vi "ConvertDocxToMDUsingWritage.vi"() -> ()   [LabVIEW 2018]
uses:
  <vilib>/regexp/Match Regular Expression.xnode
panel:
  out "FigureLabelForLink":string[](array[string])
  out "FinalOutput":string
  out "FiguresNumbers":string[](array[string])
  out "String":string
  in  "file path (use dialog)":path=path "C:/Users/jgsaenz/gitRepos/HMIComputers_documentation/00 Structure/LSST_HMI_SoftwareDocumentation_0_Structure.md"
  # "This VI mus be used after saving the docx file as md using the writage tool"
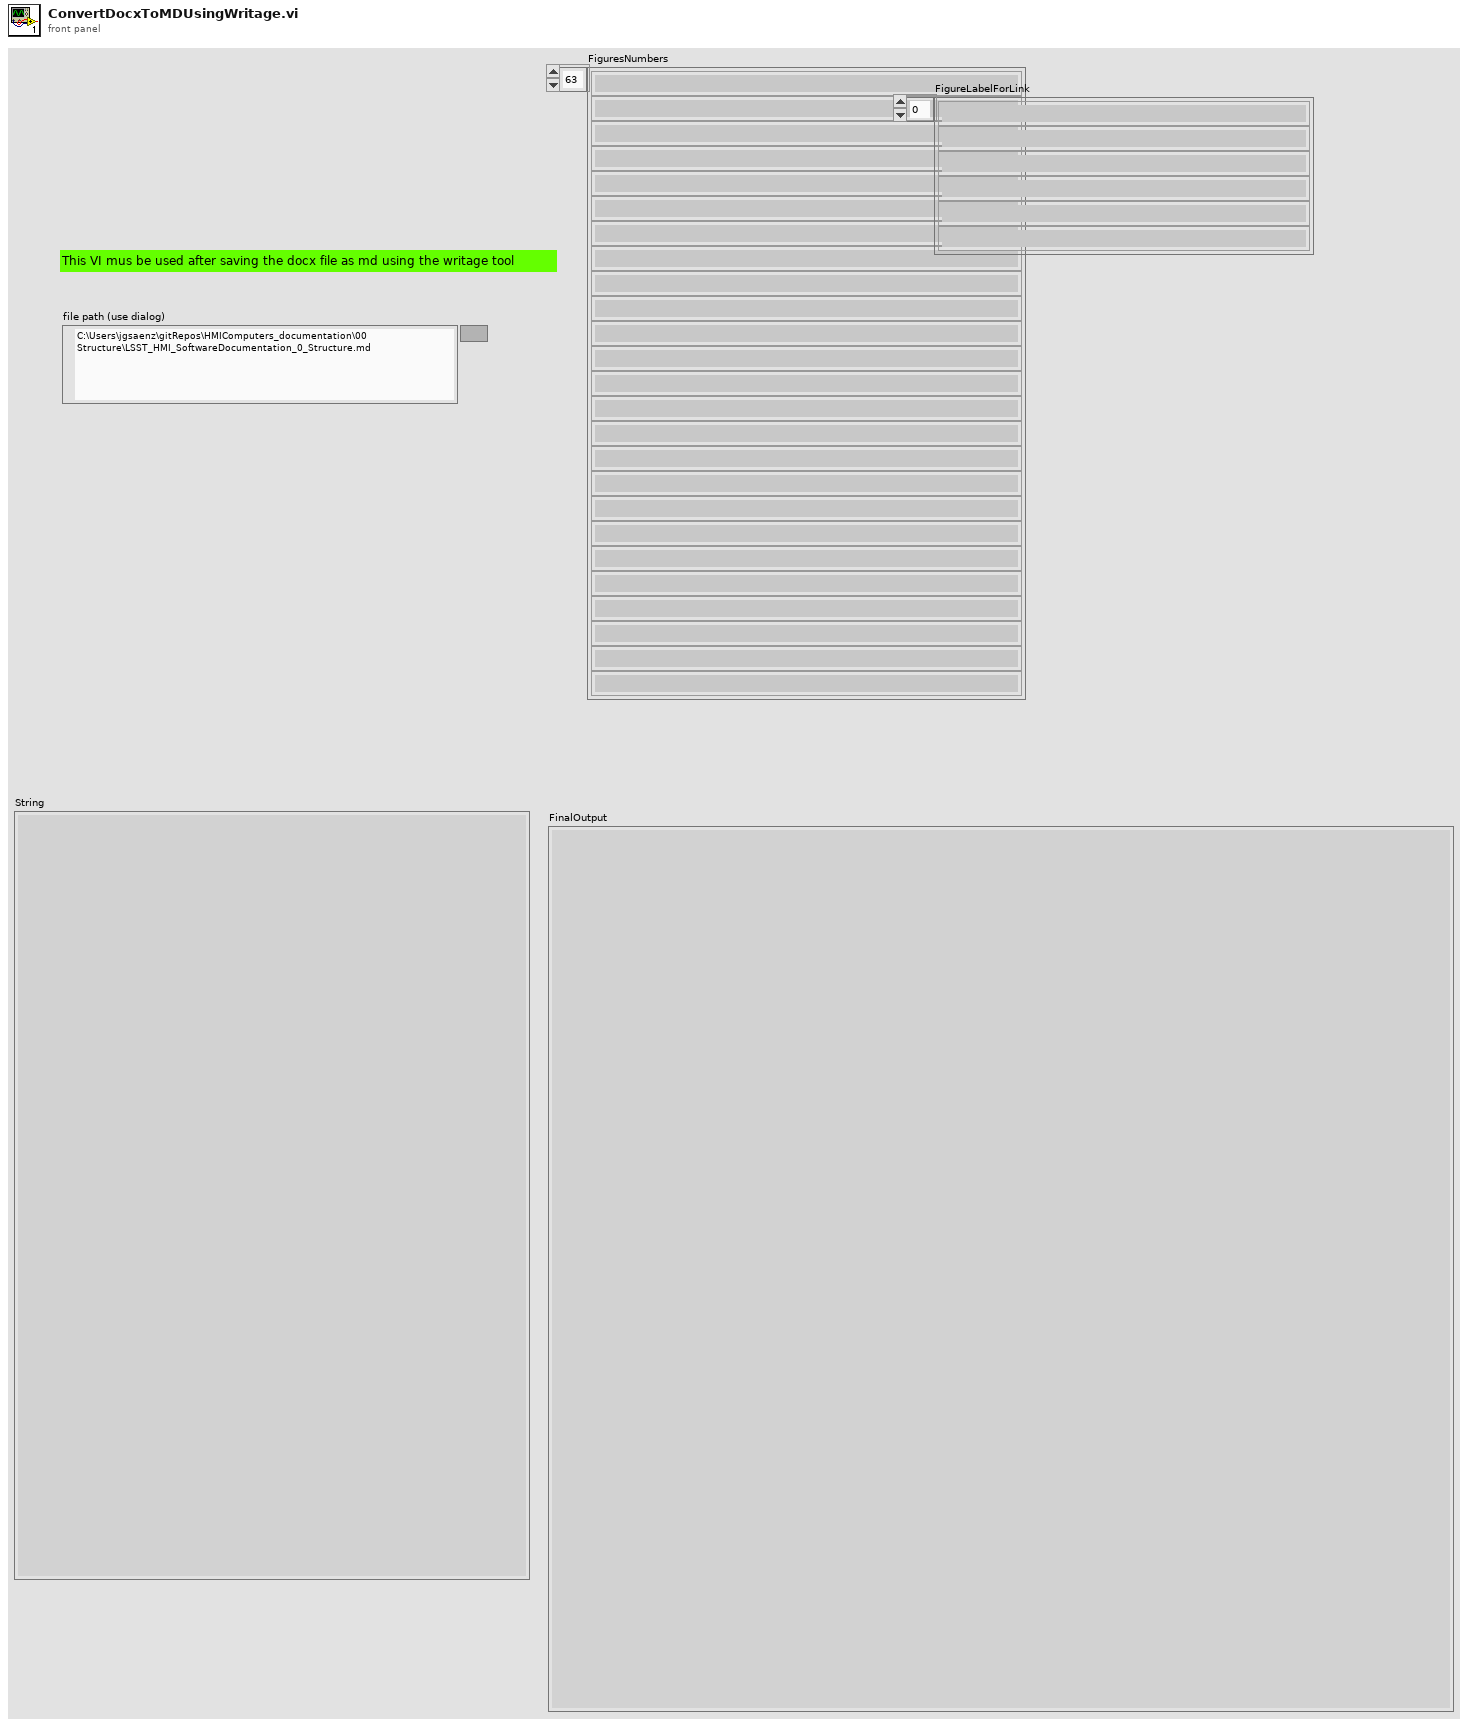
[diagram p1: front panel]
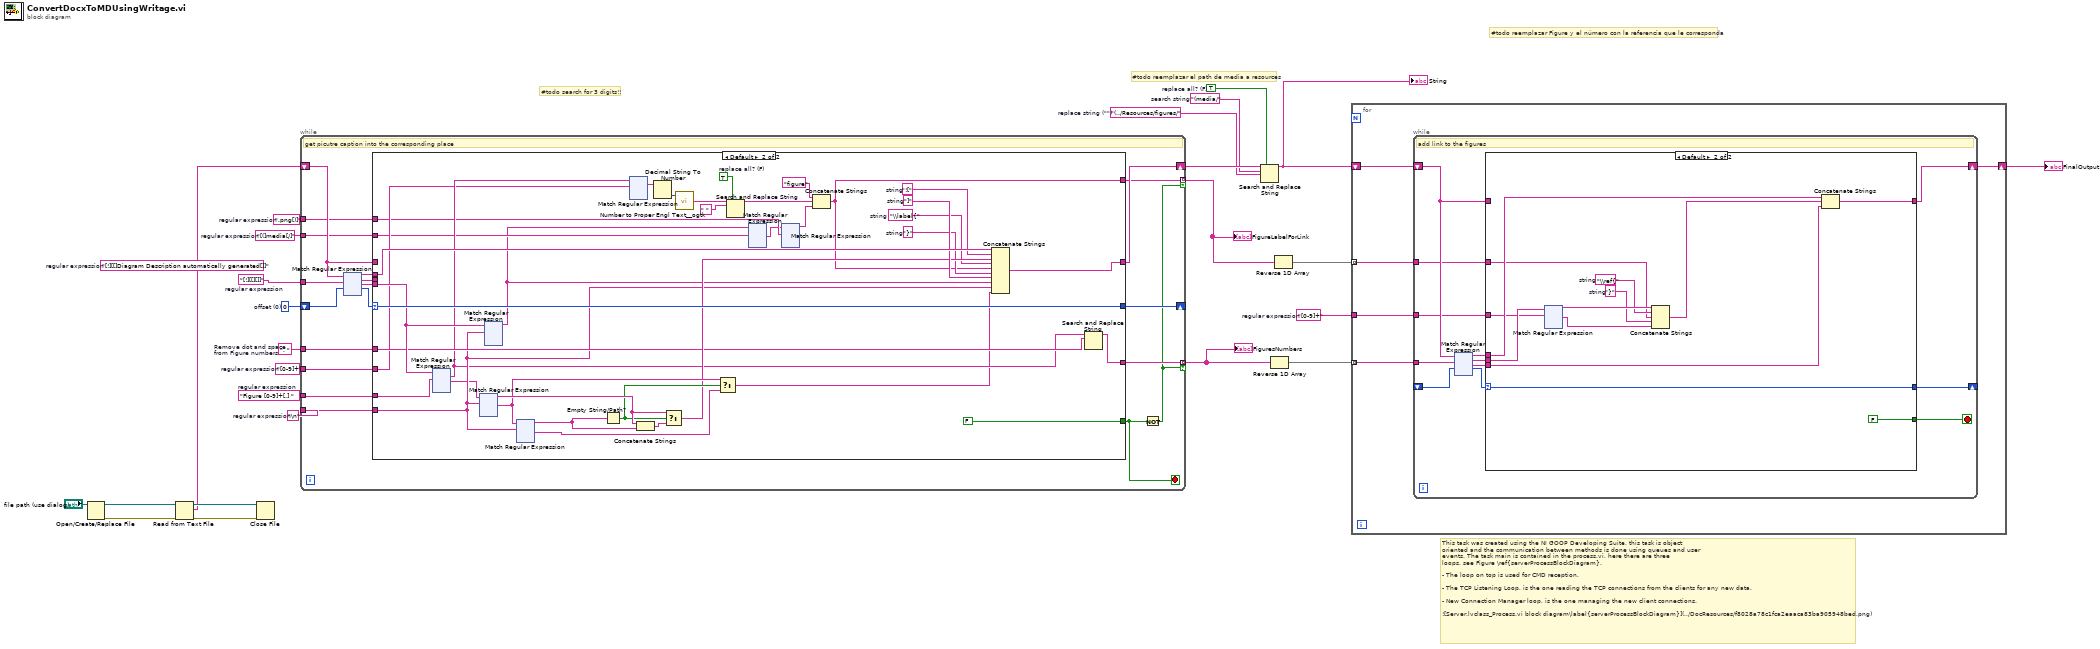
[diagram p0: block diagram]
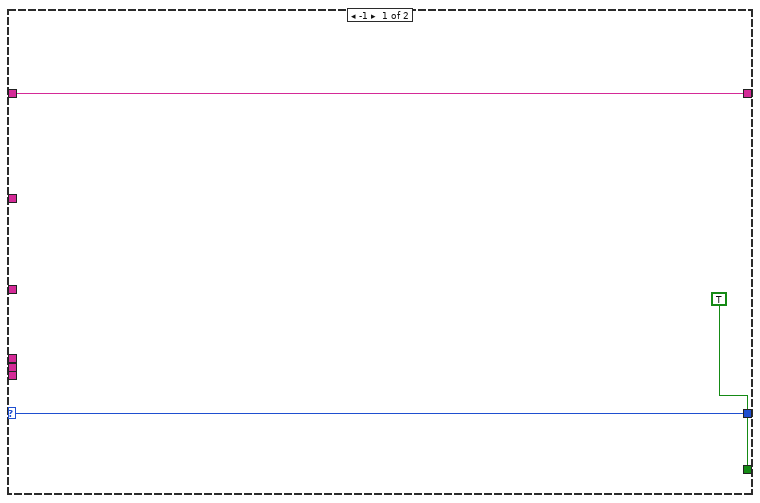
[diagram p2: hidden frame]
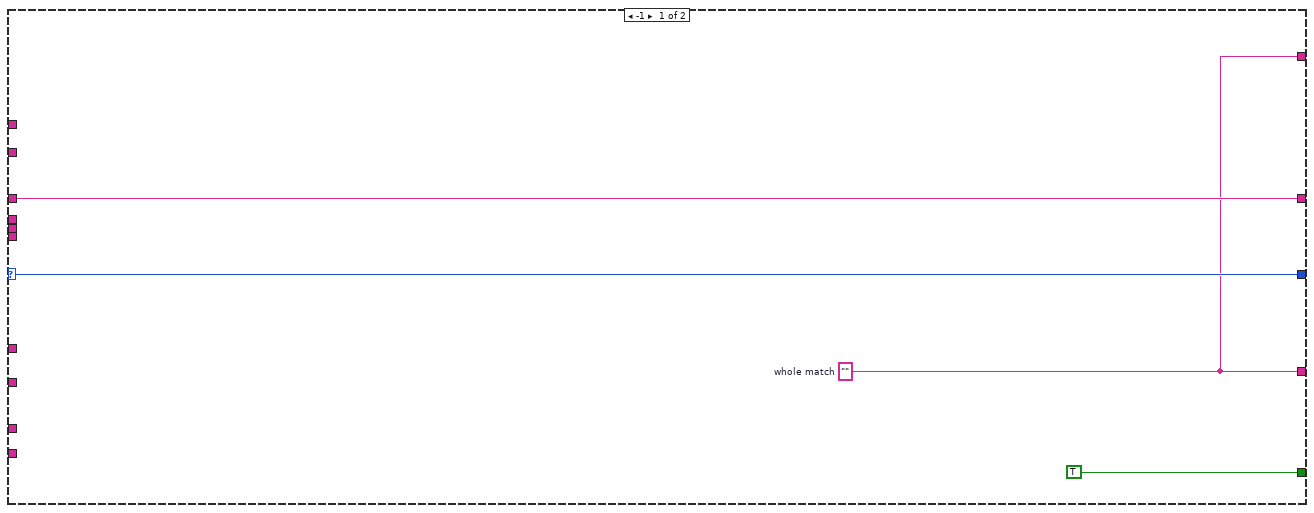
[diagram p3: hidden frame]
diagram:
  w3 = "[!][[][]]"  # regular expression
  w5 = "[0-9]+"  # regular expression
  w6 = TRUE  # replace all? (F)
  w7 = "[(]media[/]"  # regular expression
  w8 = ".png[)]"  # regular expression
  w9 = "[0-9]+"  # regular expression
  w10 = ". "  # Remove dot and space from Figure numbers
  w14 = "(../Resources/figures/"  # replace string ("")
  w15 = "(media/"  # search string
  w17 = 0  # offset (0)
  w18 = "\n"  # regular expression
  w19 = "Figure [0-9]+[.] "  # regular expression
  (unwired) "[!][[]Diagram Description automatically generated[]]"  # regular expression
  # "#todo search for 3 digits!!"
  # "#todo reemplazar el path de media a resources"
  # "#todo reemplazar Figure y el número con la referencia que le corresponda"
  # "This task was created using the NI GOOP Developing Suite, this task is object\noriented and the communication between methods is done using queues and user\nevents. The task main is contained in the process.vi, here there are three\nloops, see Figure \\ref{serverProcessBlockDiagram}.\n\n- The loop on top is used for CMD reception.\n\n- The TCP Listening Loop, is the one reading the TCP connections from the clients for any new data.\n\n- New Connection Manager loop, is the one managing the new client connections.\n\n![Server.lvclass_Process.vi block diagram\\label{serverProcessBlockDiagram}](../DocResources/f8028a78c1fca2eaaca83ba905948bed.png)"
  n1 = Open/Create/Replace File(file path (use dialog)="file path (use dialog)") -> (refnum out=w24:refnum<file>, error out=w25:errorcluster)  [unwired: 5 in, 1 out]
  n2 = Read from Text File(file (use dialog)=w24, error in=w25) -> (refnum out=w22:refnum<file>, text=w20:string, error out=w23:errorcluster)  [unwired: 2 in, 1 out]
  n3 = Close File(refnum=w22, error in=w23) -> ()  [unwired: 2 out]
  n4 = while {
    tunnel: w3 -> [w44]
    tunnel: w19 -> [w43]
    tunnel: w18 -> [w41]
    shift-right: [w38] -> _
    shift-left: w17 -> [w40]
    shift-right: [w36] -> w16
    shift-left: w20 -> [w37]
    tunnel: [w33] -> w11 mode=indexing if=w28
    tunnel: w10 -> [w31]
    tunnel: w9 -> [w30]
    tunnel: [w29] -> w4 mode=indexing if=w28
    tunnel: w8 -> [w27]
    tunnel: w7 -> [w26]
    stop <- w32 stop-if-true
    # "get picutre caption into the corresponding place"
    n5 = xnode "Match Regular Expression"("input string"=w37, "regular expression"=w44, "offset (0)"=w40) -> ("before match"=w34:string, "whole match"=w35:string, "after match"=w42:string, "offset past match"=w39:i32)  [unwired: 3 in, 1 out]
    n6 = case shown="Default" w39 {
      selector: w39 -> [w48 w81]
      tunnel: w43 -> [_ w85]
      tunnel: w42 -> [_ w75]
      tunnel: w41 -> [_ w66]
      tunnel: [w48 w81] -> w38
      tunnel: w37 -> [w47 _]
      tunnel: [w47 w79] -> w36
      tunnel: w35 -> [_ _]
      tunnel: w34 -> [_ w80]
      tunnel: [TRUE FALSE] -> w32
      tunnel: [w45 w70] -> w33
      tunnel: w31 -> [_ w69]
      tunnel: w30 -> [_ w62]
      tunnel: [w45 w60] -> w29
      tunnel: w27 -> [_ w59]
      tunnel: w26 -> [_ w55]
      frame -1 {
        w45 = ""  # whole match
      }
      frame Default {
        w50 = TRUE  # replace all? (F)
        w67 = "}"  # string
        w68 = "\\label{"  # string
        w77 = "]"  # string
        w78 = "!["  # string
        n7 = xnode "Match Regular Expression"("input string"=w75, "regular expression"=w85) -> ("whole match"=w64:string, "after match"=w57:string)  [unwired: 4 in, 3 out]
        n8 = xnode "Match Regular Expression"("input string"=w57, "regular expression"=w66) -> ("before match"=w84:string, "after match"=w73:string)  [unwired: 4 in, 3 out]
        n9 = xnode "Match Regular Expression"("input string"=w75, "regular expression"=w66) -> ("before match"=w53:string)  [unwired: 4 in, 4 out]
        n10 = xnode "Match Regular Expression"("input string"=w73, "regular expression"=w66) -> ("before match"=w82:string, "after match"=w72:string)  [unwired: 4 in, 3 out]
        n11 = Empty String/Path?(string/path=w82) -> (empty?=w74:bool)
        n12 = xnode "Match Regular Expression"("input string"=w64, "regular expression"=w62) -> ("whole match"=w63:string)  [unwired: 4 in, 4 out]
        n13 = Concatenate Strings(w84, w82) -> (w83:string)
        n14 = Decimal String To Number(string=w63) -> (number=w65:i32)  [unwired: 2 in, 1 out]
        n15 = Select(t=w84, s=w74, f=w83) -> (s? t:f=w71:string)
        n16 = call <userlib>:"Number to Proper Engl Text__ogtk.vi"("Numeric"=w65) -> ("String"=w51:string)  [unwired: 4 in]
        n17 = Select(t=w73, s=w74, f=w72) -> (s? t:f=w54:string)
        n18 = Search and Replace String(replace all?=w50, input string=w51, search string=" ") -> (result string=w52:string)  [unwired: 5 in, 3 out]
        n19 = xnode "Match Regular Expression"("input string"=w53, "regular expression"=w55) -> ("after match"=w56:string)  [unwired: 4 in, 4 out]
        n20 = xnode "Match Regular Expression"("input string"=w56, "regular expression"=w59) -> ("before match"=w58:string)  [unwired: 4 in, 4 out]
        n21 = Concatenate Strings("figure", w52, w58) -> (w60:string)
        n22 = Concatenate Strings(w80, w78, w71, w68, w60, w67, w77, w53, w66, w54) -> (w79:string)
        n23 = Search and Replace String(input string=w64, search string=w69) -> (result string=w70:string)  [unwired: 6 in, 3 out]
      }
    }
    n24 = Not(x=w32) -> (.not. x?=w28:bool)
  }
  "FiguresNumbers" <- w11
  "FigureLabelForLink" <- w4
  n25 = Search and Replace String(replace all?=w6, input string=w16, search string=w15, replace string=w14) -> (result string=w13:string)  [unwired: 4 in, 3 out]
  "String" <- w13
  n26 = Reverse 1D Array(array=w11) -> (reversed array=w2:string[])
  n27 = Reverse 1D Array(array=w4) -> (reversed array=w1:string[])
  n28 = for {
    tunnel: w2 -> [w1000] mode=indexing
    shift-right: [w1001] -> w12
    shift-left: w13 -> [w1002]
    tunnel: w5 -> [w999]
    tunnel: w1 -> [w998] mode=indexing
    n29 = while {
      tunnel: w1000 -> [w1014]
      shift-right: [w1010] -> _
      shift-left: _ -> [w1012]
      shift-right: [w1008] -> w1001
      shift-left: w1002 -> [w1009]
      tunnel: w999 -> [w1004]
      tunnel: w998 -> [w1003]
      stop <- w1005 stop-if-true
      # "add link to the figures"
      n30 = xnode "Match Regular Expression"("input string"=w1009, "regular expression"=w1014, "offset (0)"=w1012) -> ("before match"=w1006:string, "whole match"=w1007:string, "after match"=w1013:string, "offset past match"=w1011:i32)  [unwired: 3 in, 1 out]
      n31 = case shown="Default" w1011 {
        selector: w1011 -> [w1017 w1029]
        tunnel: w1013 -> [_ w1026]
        tunnel: [w1017 w1029] -> w1010
        tunnel: w1009 -> [w1015 _]
        tunnel: [w1015 w1028] -> w1008
        tunnel: w1007 -> [_ w1025]
        tunnel: w1006 -> [_ w1027]
        tunnel: [TRUE FALSE] -> w1005
        tunnel: w1004 -> [_ w1024]
        tunnel: w1003 -> [_ w1020]
        frame -1 {
        }
        frame Default {
          w1021 = "}"  # string
          w1022 = "\\ref{"  # string
          n32 = xnode "Match Regular Expression"("input string"=w1025, "regular expression"=w1024) -> ("before match"=w1023:string, "after match"=w1019:string)  [unwired: 4 in, 3 out]
          n33 = Concatenate Strings(w1023, w1022, w1020, w1021, w1019) -> (w1018:string)
          n34 = Concatenate Strings(w1027, w1018, w1026) -> (w1028:string)
        }
      }
    }
  }
  "FinalOutput" <- w12
